vi "phan_xymap.vi"() -> ()   [LabVIEW 2019]
uses:
  <vilib>/Platform/TimedLoop/XDataNode/timing_clust.ctl
  <vilib>/Platform/TimedLoop/XDataNode/nitl_modes.ctl
  <vilib>/Platform/TimedLoop/XDataNode/wakeup.ctl
  <vilib>/platform/TimedLoop/XDataNode/XDataNode.xnode
  <vilib>/Platform/TimedLoop/XDataNode/XDNodeRunTimeDep.lvlib
  <vilib>/ptbypt/NI_PtbyPt.lvlib
panel:
  in  "map 2":dbl[][](array[numeric])
  out "TOA DO 2":dbl[][](array[numeric])
  out "Ts":dbl=10.0
  out "left      right":dbl[][](array[numeric])
  out "up     down":dbl[][](array[numeric])
  out "m":i32
  out "n":i32
  out "map":dbl[][](array[numeric])
  out "i":dbl
  in  "time":dbl=2.0
  out "Vxdk":dbl
  out "Vydk":dbl
  in  "Kdv3":dbl
  in  "Kiv3":dbl=28.5
  in  "Kpv3":dbl=0.7
  in  "Kdv2":dbl
  in  "Kiv2":dbl=28.5
  in  "Kpv2":dbl=0.7
  out "sailechxy":cluster{"e_x":dbl, "e_y":dbl}(graph)
  in  "Kdxy":dbl
  in  "Kixy":dbl
  in  "Kpxy":dbl=4.0
  out "V_ph":dbl
  out "w_ph3":dbl
  out "w_ph2":dbl
  out "w_ph1":dbl
  in  "RESETMAP":bool=TRUE caption="Reset"
  out "duty3":dbl
  out "duty2":dbl
  out "duty1":dbl
  in  "RESET":bool
  out "Y_sp":dbl
  out "X_sp":dbl
  out "Y_ph":dbl
  out "X_ph":dbl
  out "Map":cluster{"Y":dbl[], "Y":dbl[]}[](graph)
  out "V3_sp":dbl
  out "V3_ph":dbl
  out "VAN TOC":T1(graph)
  in  "Kdv1":dbl
  in  "Kiv1":dbl=28.5
  in  "Kpv1":dbl=0.7
  out "V2_ph":dbl
  out "V1_ph":dbl
  out "V2_sp":dbl
  out "V1_sp":dbl
  in  "START":bool
  # "HE THONG"
  # "PID VI TRI"
  # "DUTY"
  # "PID TOC DO"
  # "TOC DO PHAN HOI (rad/s)"
  # "VI TRI DIEU KHIEN\n(m)"
  # "VI TRI PHAN HOI\n(m)"
  # "VAN TOC DIEU KHIEN\n(m/s)"
  # "VAN TOC PHAN HOI\n(m/s)"
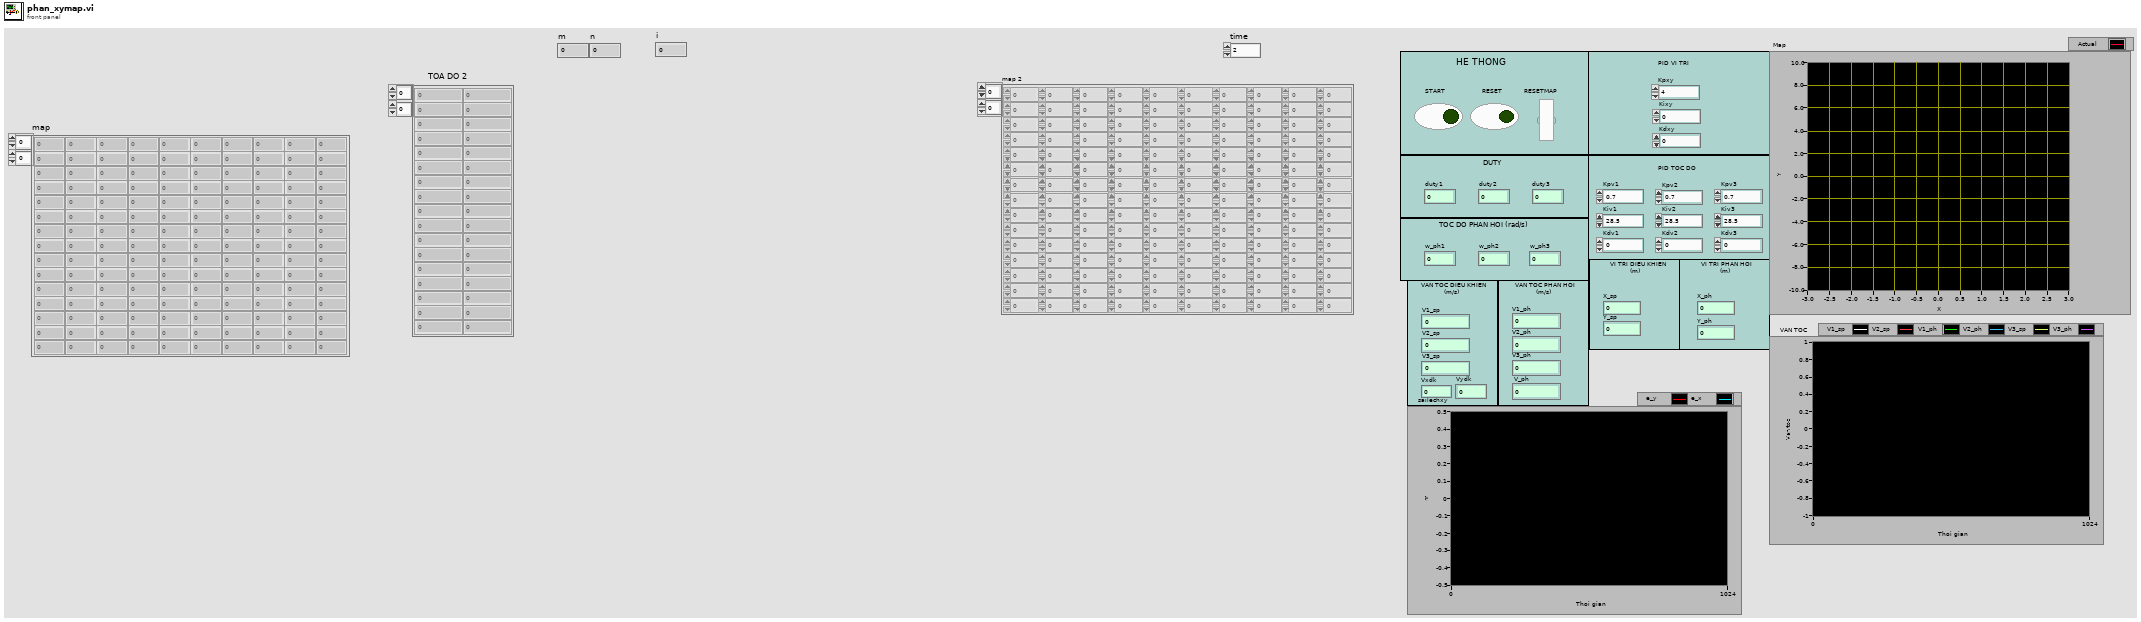
[diagram p1: front panel]
types:
  T1 = cluster{dbl, dbl, "V1_ph":dbl, "V2_ph":dbl, dbl, "V3_ph":dbl}
  T2 = typedef "XDNodeRunTimeDep.lvlib/timing_clust.ctl" = cluster{"Expected End [f-1]":u64, "Actual End [f-1]":u64, "Finished Late? [f-1]":bool, "Expected End [i-1]":u64, "Actual End [i-1]":u64, "Finished Late? [i-1]":bool, "Expected Start [i]":u64, "Actual Start [i]":u64, "Expected Start [f]":u64, "Actual Start [f]":u64, "Source Name":string, "Structure Name":string, "Period":i64, "Deadline":i64, "Offset":i64, "Start":i64, "Priority":i32, "Timeout":i32, "Mode":T3, "Wakeup Reason":T4, "Error":errorcluster, "Source Type":string, "Secondary Source Type":string, "Global End Time":u64, "Global Start Time":u64, "Frame Duration":u64, "Iteration Duration":u64, "Assigned CPU":i32, "I/O Scan Engine Mode":u32}
  T3 = typedef "XDNodeRunTimeDep.lvlib/nitl_modes.ctl" = enum32{"No Change", "Process missed periods, maintain original phase", "Discard missed periods, maintain original phase", "Process missed periods, ignore original phase", "Discard missed periods, ignore original phase"}
  T4 = typedef "XDNodeRunTimeDep.lvlib/wakeup.ctl" = enum32{"Normal", "Aborted", "Asynchronous wakeup", "Timing source error", "Timed loop error", "Timeout"}
  T5 = cluster{"V1_sp":dbl, "V_ph1":dbl, "V2_sp":dbl, "V_ph2":dbl, "V3_sp":dbl, "V_ph3":dbl}
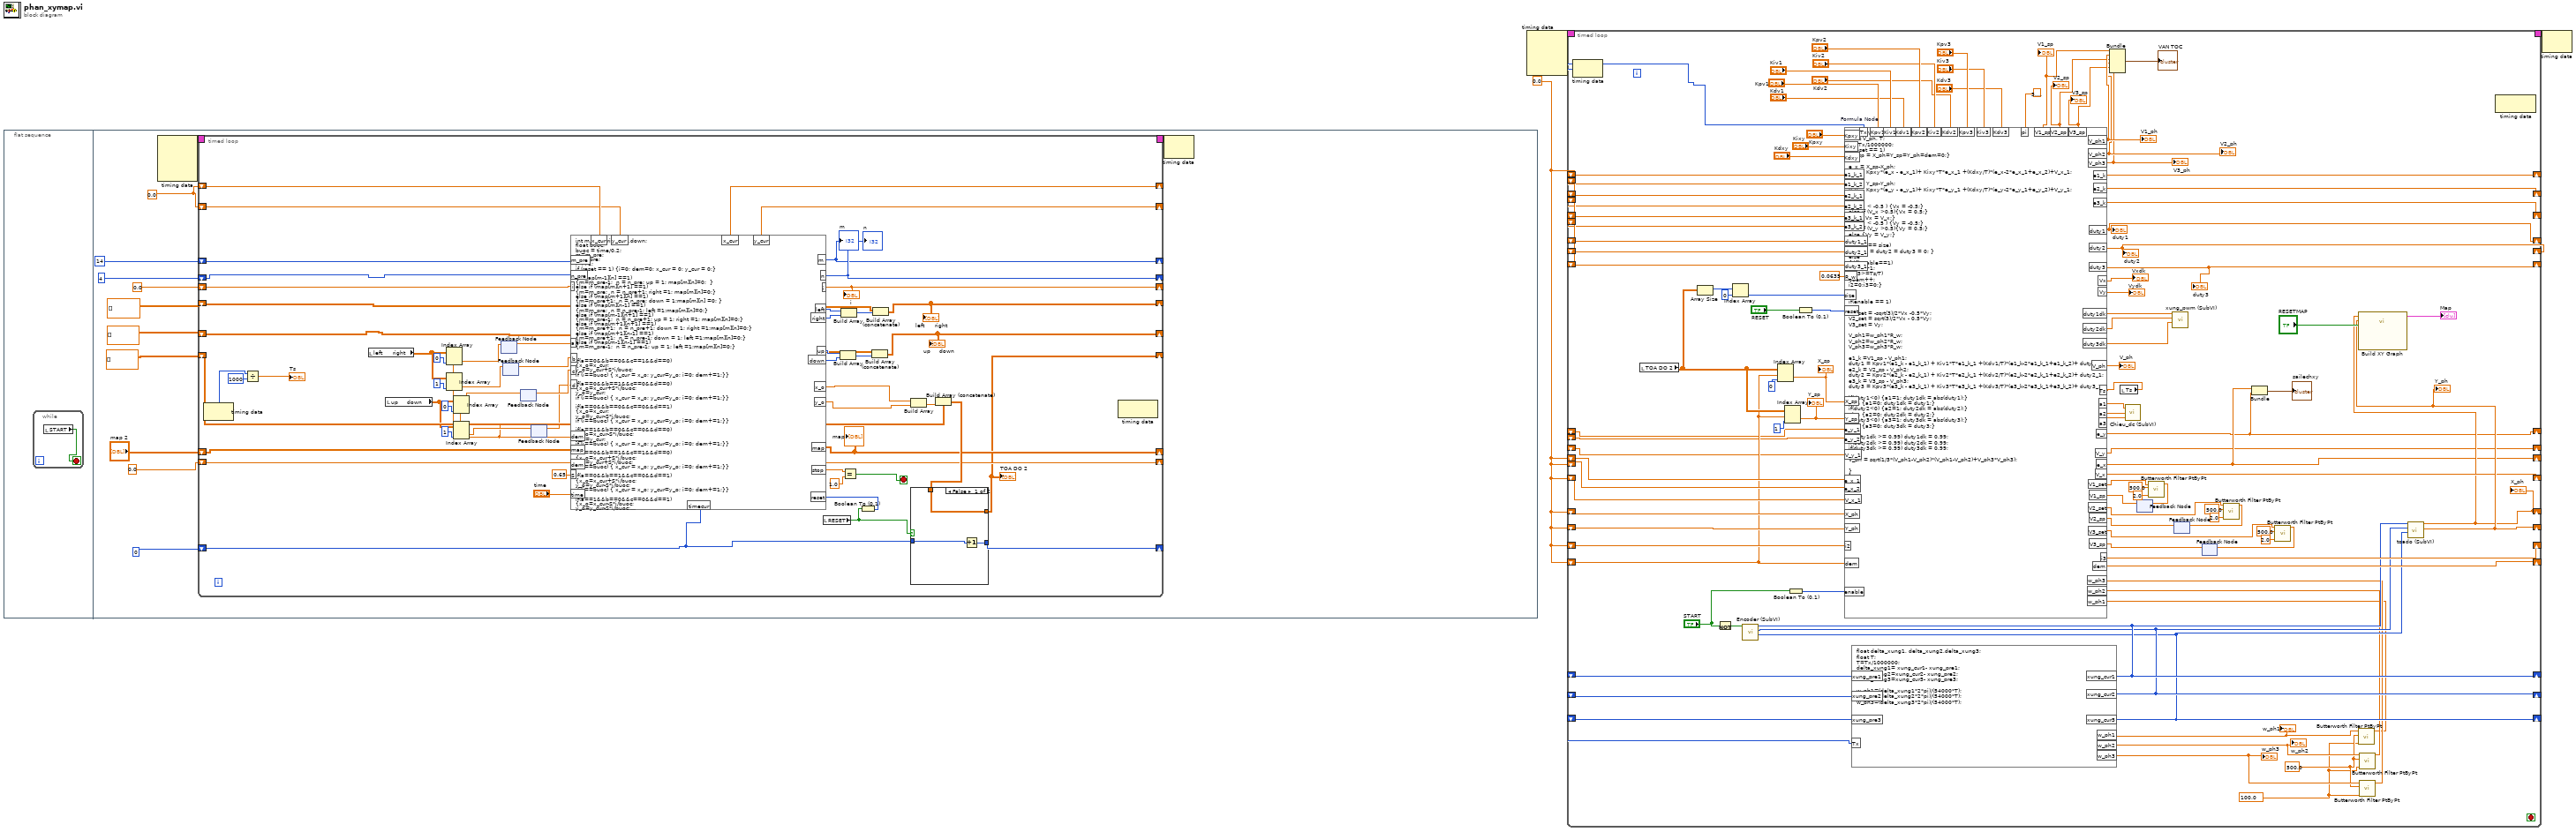
[diagram p0: block diagram]
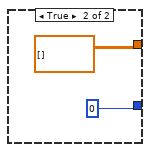
[diagram p2: hidden frame]
diagram:
  w1 = 0.0 ("e1")
  n1 = flat-sequence {
    frame #0 {
      n2 = while {
        stop <- w4 stop-if-true
        n3 = local read "START"() -> (w4:bool)
      }
    }
    frame #1 {
      w5 = 0.0 ("x_cur")
      n4 = node-c288() -> (w16:T2)  [unwired: 4 in]
      n5 = timed-loop {
        timing: w16 -> [_]
        timing-out: [_] -> w15
        shift-right: [w19] -> _
        shift-left: dbl[][] [] -> [w71]
        shift-right: [w69] -> _
        shift-left: 0 -> [w37]
        shift-right: [w28] -> _
        shift-left: 14 -> [w43]
        shift-right: [w29] -> _
        shift-left: 4 -> [w42]
        shift-right: [w31] -> _
        shift-left: dbl[][] [] -> [w40]
        shift-right: [w32] -> _
        shift-left: dbl[][] [] -> [w39]
        shift-right: [w35] -> _
        shift-left: "map 2" -> [w38]
        shift-right: [w30] -> _
        shift-left: 0.0 ("i") -> [w41]
        shift-right: [w26] -> _
        shift-left: 0.0 ("dem") -> [w27]
        shift-right: [w24] -> _
        shift-left: w5 -> [w25]
        shift-right: [w22] -> _
        shift-left: w5 -> [w23]
        stop <- w36 stop-if-true
        n6 = node-c288() -> (w68:i64)  [unwired: 1 in]
        n7 = Divide(x=w68, y=i64 1000) -> (x/y=→"Ts":dbl)
        n8 = local read "left      right"() -> (w54:dbl[][])
        n9 = local read "up     down"() -> (w18:dbl[][])
        n10 = feedback #1() -> (w50:dbl)  [unwired: 1 in]
        n11 = feedback #2() -> (w48:dbl)  [unwired: 1 in]
        n12 = feedback #3() -> (w46:dbl)  [unwired: 1 in]
        n13 = feedback #4() -> (w44:dbl)  [unwired: 1 in]
        n14 = local read "RESET"() -> (w17:bool)
        n15 = Boolean To (0,1)(Boolean=w17) -> (0, 1=w63:i16)
        n16 = formula code="int m,n,left,right,up,down;\nfloat buoc;\nbuoc = time/0.2;\nm=m_pre;\nn=n_pre;\ni=i+1;\nif (reset == 1) {i=0; dem=0; x_cur = 0; y_cur = 0;}\n\nif (map[m-1][n] ==1) \n{m=m_pre-1;  n = n_pre; up = 1; map[m][n]=0;  }\nelse if (map[m][n+1] ==1) \n{m=m_pre;  n = n_pre+1; right =1; map[m][n]=0;}\nelse if (map[m+1][n] ==1) \n{m=m_pre+1;  n = n_pre; down = 1;map[m][n] =0; }\nelse if (map[m][n-1] ==1) \n{m=m_pre;  n = n_pre-1; left =1;map[m][n]=0;}\nelse if (map[m-1][n+1] ==1) \n{m=m_pre-1;  n = n_pre+1; up = 1; right =1; map[m][n]=0;}\nelse if (map[m+1][n+1] ==1) \n{m=m_pre+1;  n = n_pre+1; down = 1; right =1;map[m][n]=0;}\nelse if (map[m+1][n-1] ==1) \n{m=m_pre+1;  n = n_pre-1; down = 1; left =1;map[m][n]=0;}\nelse if (map[m-1][n-1] ==1) \n{m=m_pre-1;  n = n_pre-1; up = 1; left =1;map[m][n]=0;}\n\n\nif(a==0&&b==0&&c==1&&d==0)\n{x_o=x_cur;\ny_o=y_cur+S*i/buoc;\nif (i==buoc) { x_cur = x_o; y_cur=y_o; i=0; dem+=1;}}\n\nif(a==0&&b==1&&c==0&&d==0)\n{x_o=x_cur+S*i/buoc;\ny_o=y_cur;\nif (i==buoc) { x_cur = x_o; y_cur=y_o; i=0; dem+=1;}}\n\nif(a==0&&b==0&&c==0&&d==1)\n{x_o=x_cur;\ny_o=y_cur-S*i/buoc;\nif (i==buoc) { x_cur = x_o; y_cur=y_o; i=0; dem+=1;}}\n\nif(a==1&&b==0&&c==0&&d==0)\n{x_o=x_cur-S*i/buoc;\ny_o=y_cur;\nif (i==buoc) { x_cur = x_o; y_cur=y_o; i=0; dem+=1;}}\n\nif(a==0&&b==1&&c==1&&d==0)\n{x_o=x_cur+S*i/buoc;\ny_o=y_cur+S*i/buoc;\nif (i==buoc) { x_cur = x_o; y_cur=y_o; i=0; dem+=1;}}\n\nif(a==0&&b==1&&c==0&&d==1)\n{x_o=x_cur+S*i/buoc;\ny_o=y_cur-S*i/buoc;\nif (i==buoc) { x_cur = x_o; y_cur=y_o; i=0; dem+=1;}}\n\nif(a==1&&b==0&&c==0&&d==1)\n{x_o=x_cur-S*i/buoc;\ny_o=y_cur-S*i/buoc;\nif (i==buoc) { x_cur = x_o; y_cur=y_o; i=0; dem+=1;}}\n\nif(a==1&&b==0&&c==1&&d==0)\n{x_o=x_cur-S*i/buoc;\ny_o=y_cur+S*i/buoc;\nif (i==buoc) { x_cur = x_o; y_cur=y_o; i=0; dem+=1;}}"("timecur"=w37, "map"=w38, "reset"=w63, "m_pre"=w43, "n_pre"=w42, "i"=w41, "a"=w50, "b"=w48, "c"=w46, "d"=w44, "dem"=w27, "x_cur"=w25, "y_cur"=w23, "time"="time", "S"=0.65 ("input variable")) -> ("x_o"=w34:dbl, "y_o"=w33:dbl, "stop"=w65:dbl, "m"=w28:i32, "n"=w29:i32, "left"=w62:i32, "right"=w61:i32, "up"=w60:i32, "down"=w59:i32, "map"=w35:dbl[][], "i"=w30:dbl, "dem"=w26:dbl, "x_cur"=w24:dbl, "y_cur"=w22:dbl)
        "m" <- w28
        "n" <- w29
        "map" <- w35
        "i" <- w30
        n17 = Index Array(array=w54, index (row)=w26, index (col)=0 ("disabled index (col)")) -> (element=w51:dbl)
        n18 = Index Array(array=w54, index (row)=w26, index (col)=1 ("disabled index (col)")) -> (element=w49:dbl)
        n19 = Index Array(array=w18, index (row)=w26, index (col)=0 ("disabled index (col)")) -> (element=w47:dbl)
        n20 = Index Array(array=w18, index (row)=w26, index (col)=1 ("disabled index (col)")) -> (element=w45:dbl)
        n21 = feedback-in #1(w51) -> ()
        n22 = feedback-in #2(w49) -> ()
        n23 = feedback-in #3(w47) -> ()
        n24 = feedback-in #4(w45) -> ()
        n25 = Build Array(w60, w59) -> (w57:i32[])
        n26 = Build Array(w62, w61) -> (w58:i32[])
        n27 = Equal?(x=w65, y=1.0) -> (x = y?=w36:bool)
        n28 = Build Array (concatenate)(w39, w57) -> (w32:dbl[][])
        "up     down" <- w32
        n29 = Build Array (concatenate)(w40, w58) -> (w31:dbl[][])
        "left      right" <- w31
        n30 = Build Array(w34, w33) -> (w72:dbl[])
        n31 = Build Array (concatenate)(w71, w72) -> (w70:dbl[][])
        n32 = case shown="False" w17 {
          tunnel: w70 -> [w75 _]
          tunnel: [w75 dbl[][] []] -> w19
          tunnel: [w74 0] -> w69
          tunnel: w37 -> [w73 _]
          frame False {
            n33 = Increment(x=w73) -> (x+1=w74:i32)
          }
          frame True {
          }
        }
        "TOA DO 2" <- w19
        n34 = node-c288() -> ()  [unwired: 1 in, 1 out]
      }
      n35 = node-c288(w15) -> ()  [unwired: 1 out]
    }
  }
  n36 = node-c288() -> (w3:T2)  [unwired: 4 in]
  n37 = timed-loop {
    timing: w3 -> [_]
    timing-out: [_] -> w2
    shift-right: [w192] -> _
    shift-left: w1 -> [w190]
    shift-right: [w191] -> _
    shift-left: w1 -> [w143]
    shift-right: [w183] -> _
    shift-left: w1 -> [w182]
    shift-right: [w110] -> _
    shift-left: w1 -> [w181]
    shift-right: [w160] -> _
    shift-left: w1 -> [w180]
    shift-right: [w179] -> _
    shift-left: w1 -> [w111]
    shift-right: [w158] -> _
    shift-left: w1 -> [w159]
    shift-right: [w157] -> _
    shift-left: w1 -> [w154]
    shift-right: [w156] -> _
    shift-left: w1 -> [w153]
    shift-right: [w155] -> _
    shift-left: w1 -> [w152]
    shift-right: [w146] -> _
    shift-left: _ -> [w149]
    shift-right: [w145] -> _
    shift-left: _ -> [w148]
    shift-right: [w144] -> _
    shift-left: _ -> [w147]
    shift-right: [w93] -> _
    shift-left: w1 -> [w138]
    shift-right: [w136] -> _
    shift-left: w1 -> [w137]
    shift-left: w1 -> [w132]
    shift-left: w1 -> [w131]
    shift-left: w1 -> [w130]
    shift-left: w1 -> [w129]
    shift-right: [w84] -> _
    shift-left: _ -> [w89]
    shift-right: [w91] -> _
    shift-left: _ -> [w90]
    shift-left: _ -> [w88]
    stop <- _ stop-if-true
    w123 = 100.0 ("flw")
    w124 = 500.0 ("sampling freq: fs")
    n38 = node-c288() -> (w83:i64)  [unwired: 1 in]
    n39 = local read "TOA DO 2"() -> (w112:dbl[][])
    n40 = Array Size(array=w112) -> (size(s)=w175:i32[])
    n41 = Not(x="START") -> (.not. x?=w162:bool)
    n42 = Index Array(array=w175, index=0) -> (element=w173:i32)
    n43 = call "Encoder (SubVI).vi"("Boolean"=w162) -> ("Counter Value3"=w144:i32, "Counter Value 2"=w145:i32, "Counter Value"=w146:i32)  [unwired: 8 in]
    n44 = Index Array(array=w112, index (row)=w111, index (col)=0 ("disabled index (col)")) -> (element=w177:dbl)
    "X_sp" <- w177
    n45 = Index Array(array=w112, index (row)=w111, index (col)=1 ("disabled index (col)")) -> (element=w176:dbl)
    "Y_sp" <- w176
    n46 = Boolean To (0,1)(Boolean="START") -> (0, 1=w189:i16)
    n47 = Boolean To (0,1)(Boolean="RESET") -> (0, 1=w172:i16)
    n48 = formula code="float delta_xung1, delta_xung2,delta_xung3;\nfloat T; \nT=Tx/1000000;\ndelta_xung1= xung_cur1- xung_pre1;\ndelta_xung2=xung_cur2- xung_pre2;\ndelta_xung3=xung_cur3- xung_pre3; \n\nw_ph1=(delta_xung1*2*pi)/(54000*T);\nw_ph2=(delta_xung2*2*pi)/(54000*T);\nw_ph3=(delta_xung3*2*pi)/(54000*T);"("xung_pre1"=w149, "xung_pre2"=w148, "xung_pre3"=w147, "xung_cur1"=w146, "xung_cur2"=w145, "xung_cur3"=w144, "Tx"=w83) -> ("w_ph1"=w114:dbl, "w_ph2"=w126:dbl, "w_ph3"=w125:dbl)
    "w_ph1" <- w114
    "w_ph2" <- w126
    "w_ph3" <- w125
    n49 = local read "Ts"() -> (w85:dbl)
    n50 = feedback #5() -> (w101:dbl)  [unwired: 1 in]
    n51 = feedback #6() -> (w98:dbl)  [unwired: 1 in]
    n52 = feedback #7() -> (w95:dbl)  [unwired: 1 in]
    n53 = call <vilib>:"Butterworth Filter PtByPt.vi"("low cutoff freq: fl"=w123, "sampling freq: fs"=w124, "x"=w114) -> ("Filtered x"=w113:dbl)  [unwired: 6 in, 1 out]
    n54 = call <vilib>:"Butterworth Filter PtByPt.vi"("low cutoff freq: fl"=w123, "sampling freq: fs"=w124, "x"=w126) -> ("Filtered x"=w122:dbl)  [unwired: 6 in, 1 out]
    n55 = call <vilib>:"Butterworth Filter PtByPt.vi"("low cutoff freq: fl"=w123, "sampling freq: fs"=w124, "x"=w125) -> ("Filtered x"=w121:dbl)  [unwired: 6 in, 1 out]
    n56 = formula code="float V,Vtest, S_sp, S_ph, Vx, Vy;\nfloat V_ph, T;\n T=Tx/1000000;\nif(reset == 1)\n{X_sp = X_ph=Y_sp=Y_ph=dem=0;}\n\ne_x = X_sp-X_ph; \nV_x = Kpxy*(e_x - e_x_1)+ Kixy*T*e_x_1 +(Kdxy/T)*(e_x-2*e_x_1+e_x_2)+V_x_1;\n\ne_y = Y_sp-Y_ph; \nV_y = Kpxy*(e_y - e_y_1)+ Kixy*T*e_y_1 +(Kdxy/T)*(e_y-2*e_y_1+e_y_2)+V_y_1;\n\n\nif (V_x < -0.5 ) {Vx = -0.5;} \nelse if (V_x >0.5){Vx = 0.5;}\nelse {Vx = V_x;}\nif (V_y < -0.5 ) {Vy = -0.5;} \nelse if (V_y >0.5){Vy = 0.5;}\nelse {Vy = V_y;}\n\nif(dem == size)\n{duty1 = duty2 = duty3 = 0; }\nelse\n{ if(enable==1)\n i3=i2+1;\nif (i3>=Ts/T)\n{dem++;\ni2=0;i3=0;}\n\n\nif(enable == 1)\n{\nV1_set = -sqrt(3)/2*Vx -0.5*Vy;\nV2_set = sqrt(3)/2*Vx - 0.5*Vy;\nV3_set = Vy; \n\nV_ph1=w_ph1*R_w;\nV_ph2=w_ph2*R_w;\nV_ph3=w_ph3*R_w;\n\ne1_k =V1_sp - V_ph1;\nduty1 = Kpv1*(e1_k - e1_k_1) + Kiv1*T*e1_k_1 +(Kdv1/T)*(e1_k-2*e1_k_1+e1_k_2)+ duty1_1;\ne2_k = V2_sp - V_ph2;\nduty2 = Kpv2*(e2_k - e2_k_1) + Kiv2*T*e2_k_1 +(Kdv2/T)*(e2_k-2*e2_k_1+e2_k_2)+ duty2_1;\ne3_k = V3_sp - V_ph3;\nduty3 = Kpv3*(e3_k - e3_k_1) + Kiv3*T*e3_k_1 +(Kdv3/T)*(e3_k-2*e3_k_1+e3_k_2)+ duty3_1;\n\nif(duty1<0) {a1=1; duty1dk = abs(duty1);}\nelse {a1=0; duty1dk = duty1;}\nif(duty2<0) {a2=1; duty2dk = abs(duty2);}\nelse {a2=0; duty2dk = duty2;}\nif(duty3<0) {a3=1; duty3dk = abs(duty3);}\nelse {a3=0; duty3dk = duty3;}\n\nif(duty1dk >= 0.99) duty1dk = 0.99;\nif(duty2dk >= 0.99) duty2dk = 0.99;\nif(duty3dk >= 0.99) duty3dk = 0.99;\n\nV_ph = sqrt(1/3*(V_ph1-V_ph2)*(V_ph1-V_ph2)+V_ph3*V_ph3);\n\n}\n}"("Kpv1"="Kpv1", "Kiv1"="Kiv1", "Kdv1"="Kdv1", "pi"=3.141592653589793, "e1_k_1"=w190, "e2_k_1"=w143, "enable"=w189, "Tx"=w83, "e3_k_1"=w182, "X_ph"=w181, "X_sp"=w177, "Y_sp"=w176, "Y_ph"=w180, "dem"=w111, "size"=w173, "reset"=w172, "i2"=w159, "duty1_1"=w154, "duty2_1"=w153, "duty3_1"=w152, "w_ph1"=w113, "w_ph2"=w122, "w_ph3"=w121, "e_x_1"=w138, "V_x_1"=w137, "Kpxy"="Kpxy", "Kixy"="Kixy", "Kdxy"="Kdxy", "e1_k_2"=w132, "e2_k_2"=w131, "e3_k_2"=w130, "e_x_2"=w129, "Ts"=w85, "Kpv2"="Kpv2", "Kiv2"="Kiv2", "Kdv2"="Kdv2", "Kpv3"="Kpv3", "Kiv3"="Kiv3", "Kdv3"="Kdv3", "V1_sp"=w101, "V2_sp"=w98, "V3_sp"=w95, "R_w"=0.0635 ("input variable"), "e_y_1"=w89, "e_y_2"=w88, "V_y_1"=w90) -> ("V1_sp"=w170:dbl, "V_ph1"=w169:dbl, "V_ph2"=w167:dbl, "e1_k"=w192:dbl, "e2_k"=w191:dbl, "V2_sp"=w168:dbl, "duty1"=w157:dbl, "duty2"=w156:dbl, "e3_k"=w183:dbl, "V_ph3"=w166:dbl, "V3_sp"=w165:dbl, "duty3"=w155:dbl, "a1"=w161:dbl, "a2"=w151:dbl, "a3"=w150:dbl, "dem"=w179:dbl, "i3"=w158:dbl, "duty1dk"=w142:dbl, "duty2dk"=w141:dbl, "duty3dk"=w140:dbl, "V_ph"=→"V_ph":dbl, "e_x"=w93:dbl, "V_x"=w136:dbl, "V1_set"=w103:dbl, "V2_set"=w100:dbl, "V3_set"=w97:dbl, "e_y"=w84:dbl, "V_y"=w91:dbl, "Vx"=→"Vxdk":dbl, "Vy"=→"Vydk":dbl)
    "V1_sp" <- w170
    "V2_sp" <- w168
    "V1_ph" <- w169
    "V2_ph" <- w167
    "V3_ph" <- w166
    "V3_sp" <- w165
    "duty1" <- w157
    "duty2" <- w156
    "duty3" <- w155
    n57 = Bundle("V1_sp"=w170, "V_ph1"=w169, "V2_sp"=w168, "V_ph2"=w167, "V3_sp"=w165, "V_ph3"=w166) -> (→"VAN TOC":T5)  [unwired: 1 in]
    n58 = call "Chieu_dc (SubVI).vi"("a3"=w150, "a2"=w151, "a1"=w161) -> ()
    n59 = call <vilib>:"Butterworth Filter PtByPt.vi"("low cutoff freq: fl"=2.0, "sampling freq: fs"=500.0, "x"=w103) -> ("Filtered x"=w102:dbl)  [unwired: 6 in, 1 out]
    n60 = feedback-in #5(w102) -> ()
    n61 = call "xung_pwm (SubVI).vi"("duty3 in"=w140, "duty2 in"=w141, "duty1 in"=w142) -> ()  [unwired: 6 in, 3 out]
    n62 = call <vilib>:"Butterworth Filter PtByPt.vi"("low cutoff freq: fl"=2.0, "sampling freq: fs"=500.0, "x"=w100) -> ("Filtered x"=w99:dbl)  [unwired: 6 in, 1 out]
    n63 = feedback-in #6(w99) -> ()
    n64 = Bundle("e_x"=w93, "e_y"=w84) -> (→"sailechxy":cluster{"e_x":dbl, "e_y":dbl})  [unwired: 1 in]
    n65 = call <vilib>:"Butterworth Filter PtByPt.vi"("low cutoff freq: fl"=2.0, "sampling freq: fs"=500.0, "x"=w97) -> ("Filtered x"=w96:dbl)  [unwired: 6 in, 1 out]
    n66 = feedback-in #7(w96) -> ()
    n67 = call "toado (SubVI).vi"("X3"=w144, "X2"=w145, "X1"=w146) -> ("Y_ph"=w160:dbl, "X_ph"=w110:dbl)  [unwired: 7 in]
    "X_ph" <- w110
    "Y_ph" <- w160
    n68 = call "Build XY Graph"("Reset"="RESETMAP", "Y Input"=w160, "X Input"=w110) -> ("XY Graph"=→"Map":cluster{"X":dbl[], "Y":dbl[]}[])  [unwired: 7 in, 1 out]
    n69 = node-c288() -> ()  [unwired: 1 in, 1 out]
  }
  n70 = node-c288(w2) -> ()  [unwired: 1 out]
